vi "NT_CreateInstance.vi"(8 "error in (no error)":errorcluster) -> (0 "error out":errorcluster, 3 "InstanceHandle":u64)   [LabVIEW 2025]
uses:
  FRC_NetworkTablesLV.dll
  ntcoreffi.dll
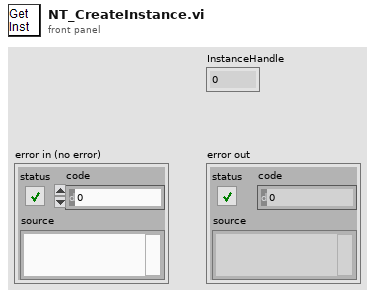
[diagram p1: front panel]
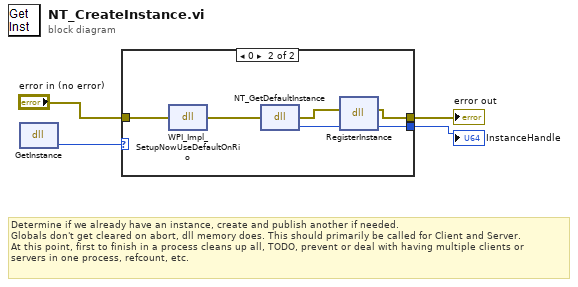
[diagram p0: block diagram]
diagram:
  # "Determine if we already have an instance, create and publish another if needed.\nGlobals don't get cleared on abort, dll memory does. This should primarily be called for Client and Server.\nAt this point, first to finish in a process cleans up all, TODO, prevent or deal with having multiple clients or\nservers in one process, refcount, etc."
  n1 = dll-call lib="FRC_NetworkTablesLV.*" fn="GetInstance"() -> ("InstanceHandle"=w4:u64)  [unwired: 3 in, 2 out]
  n2 = case shown="0" w4 {
    selector: w4 -> [w5 _]
    tunnel: [w5 w9] -> w1
    tunnel: [w6 w10] -> w2
    tunnel: "error in (no error)" -> [w6 w8]
    frame Default {
    }
    frame 0 {
      n3 = dll-call lib="ntcoreffi.*" fn="WPI_Impl_SetupNowUseDefaultOnRio"(error in=w8) -> (error out=w7:errorcluster)  [unwired: 3 in, 1 out]
      n4 = dll-call lib="ntcoreffi.*" fn="NT_GetDefaultInstance"(error in=w7) -> (error out=w11:errorcluster, "InstanceHandle"=w9:u32)  [unwired: 2 in, 1 out]
      n5 = dll-call lib="FRC_NetworkTablesLV.*" fn="RegisterInstance"(error in=w11, "inst"=w9) -> (error out=w10:errorcluster)  [unwired: 4 in, 1 out]
    }
  }
  "error out" <- w2
  "InstanceHandle" <- w1
